vi "Dead band vi by ben.vi"(10 "Numeric":dbl format="%#_13g") -> (2 "Deadbanded Value":dbl format="%#_13g")   [LabVIEW 2020]
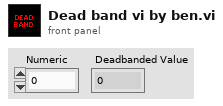
[diagram p1: front panel]
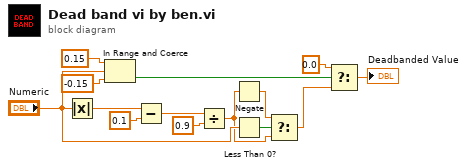
[diagram p0: block diagram]
diagram:
  n1 = Absolute Value(x="Numeric") -> (abs(x)=w11:dbl)
  n2 = In Range and Coerce(upper limit=0.15, x="Numeric", lower limit=-0.15) -> (In Range?=w3:bool)  [unwired: 1 out]
  n3 = Subtract(x=w11, y=0.1) -> (x-y=w9:dbl)
  n4 = Divide(x=w9, y=0.9) -> (x/y=w6:dbl)
  n5 = Negate(x=w6) -> (-x=w7:dbl)
  n6 = Less Than 0?(x="Numeric") -> (x < 0?=w2:bool)
  n7 = Select(t=w7, s=w2, f=w6) -> (s? t:f=w5:dbl)
  n8 = Select(t=0.0, s=w3, f=w5) -> (s? t:f=→"Deadbanded Value":dbl)
